vi "configure.vi"(0 "Imaging in":refnum<class "Imaging.lvclass">, 5 "Frame Rate":dbl, 7 "Save Flag Reference":refnum<vi>, 9 "Exposure":dbl, 11 "error in (no error)":errorcluster, 12 "Gain":dbl, 14 "Codec":string) -> (4 "Imaging out":refnum<class "Imaging.lvclass">, 15 "error out":errorcluster)   [LabVIEW 2014, in "Imaging.lvclass"]
uses:
  Imaging.lvclass
  <resource>/objmgr/IMAQImage.rc
  <vilib>/vision/driver/NI_Vision_Acquisition_Software.lvlib
  <vilib>/vision/driver/IMAQdx.llb/IMAQdx Acquisition Mode.ctl
  <vilib>/vision/driver/IMAQdx.llb/IMAQdx Buffer Number Mode.ctl
  <vilib>/vision/Image Controls.llb/IMAQ Image.ctl
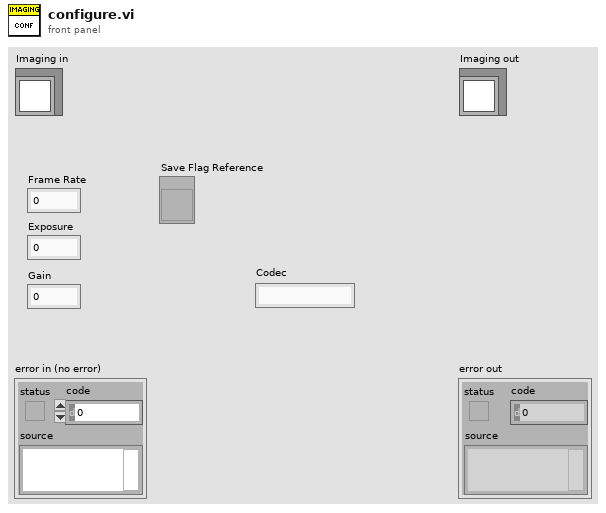
[diagram p1: front panel]
types:
  T1 = typedef "IMAQ Image.ctl" = refnum<image>
  T2 = cluster{"Image Out":T1, dbl, "seconds since 1Jan1904":timestamp}
  T3 = typedef "NI_Vision_Acquisition_Software.lvlib/IMAQdx Buffer Number Mode.ctl" = enum32{"Next", "Last", "Buffer Number", "Every", "Last New"}
  T4 = typedef "NI_Vision_Acquisition_Software.lvlib/IMAQdx Acquisition Mode.ctl" = enum32{"One Shot", "Continuous"}
  T5 = typedef "IMAQdx.ctl" = refnum<k21>
  T6 = typedef "NI_Vision_Acquisition_Software.lvlib/IMAQdx Attribute Type.ctl" = enum32{"U32", "I64", "DBL", "String", "Enum", "Bool", "Command"}
  T7 = cluster{"Attribute Type":T6, "Readable":bool, "Writable":bool, "Attribute Name":string}[]
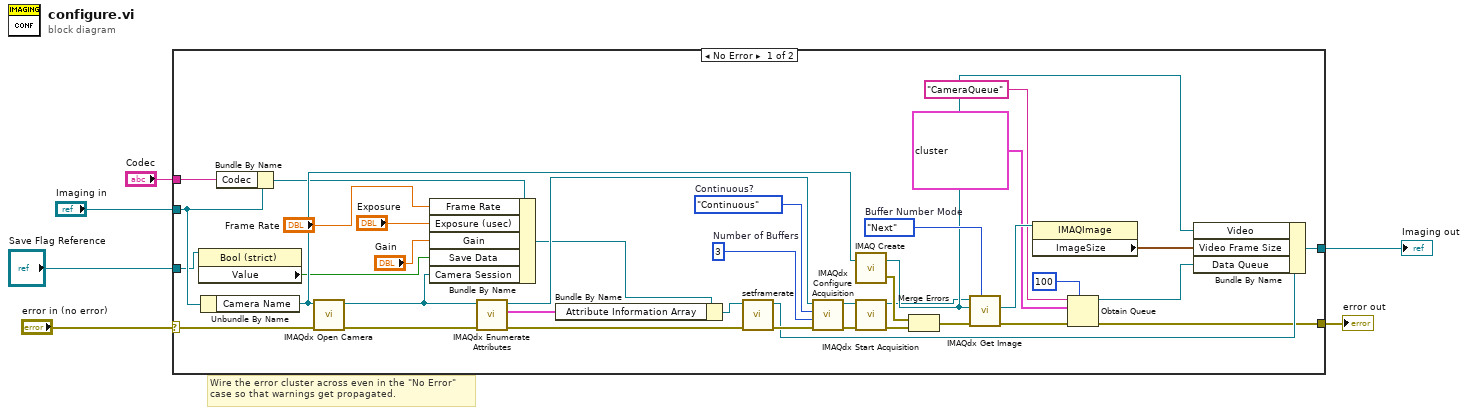
[diagram p0: block diagram]
diagram:
  # "Wire the error cluster across even in the \"No Error\"\ncase so that warnings get propagated."
  n1 = case shown="No Error" "error in (no error)" {
    selector: "error in (no error)" -> [w37 w46]
    tunnel: [w9 w46] -> w5
    tunnel: [w10 w45] -> w3
    tunnel: "Imaging in" -> [w26 w45]
    tunnel: "Codec" -> [w11 _]
    tunnel: "Save Flag Reference" -> [w7 _]
    frame No Error {
      w39 = IMAQdx_Buffer_Number_Mode."Next"  # Buffer Number Mode
      w43 = u32 3  # Number of Buffers
      w44 = IMAQdx_Acquisition_Mode."Continuous"  # Continuous?
      n2 = property class="Bool (strict)"(reference=w7) -> ("Value"=w8:bool)  [unwired: 1 in, 2 out]
      n3 = Unbundle By Name(w26) -> ("Camera Name"=w38:T5)
      n4 = Bundle By Name(cluster=w26, "Codec"=w11) -> (w25:refnum<class "Imaging.lvclass">)
      n5 = call <vilib>:"IMAQdx Open Camera.vi"("error in"=w37, "Session In"=w38) -> ("error out"=w29:errorcluster, "Session Out"=w23:T5)  [unwired: 1 in, 7 out]
      n6 = Bundle By Name(cluster=w25, "Frame Rate"="Frame Rate", "Exposure (usec)"="Exposure", "Gain"="Gain", "Save Data"=w8, "Camera Session"=w23) -> (w20:refnum<class "Imaging.lvclass">)
      n7 = call <vilib>:"IMAQdx Enumerate Attributes.vi"("error in"=w29, "Session In"=w23) -> ("error out"=w18:errorcluster, "Attribute Information Array"=w28:T7, "Session Out"=w21:T5)  [unwired: 7 in]
      n8 = Bundle By Name(cluster=w20, "Attribute Information Array"=w28) -> (w17:refnum<class "Imaging.lvclass">)
      n9 = call-dynamic "setframerate.vi"("error in (no error)"=w18, "Imaging in"=w17) -> ("error out"=w16:errorcluster, "Imaging out"=w15:refnum<class "Imaging.lvclass">)  [unwired: 8 in]
      n10 = call <vilib>:"IMAQdx Configure Acquisition.vi"("error in"=w16, "Number of Buffers"=w43, "Continuous?"=w44, "Session In"=w21) -> ("error out"=w22:errorcluster, "Session Out"=w24:T5)  [unwired: 6 out]
      n11 = call "IMAQ Create"("Image Name"=w38) -> ("New Image"=w36:T1, "error out"=w42:errorcluster)  [unwired: 3 in, 1 out]
      n12 = call <vilib>:"IMAQdx Start Acquisition.vi"("error in"=w22, "Session In"=w24) -> ("error out"=w41:errorcluster, "Session Out"=w19:T5)  [unwired: 8 out]
      n13 = Merge Errors(w42, w41) -> (w14:errorcluster)
      n14 = call <vilib>:"IMAQdx Get Image.vi"("Buffer Number Mode (Next)"=w39, "error in"=w14, "Image In"=w36, "Session In"=w19) -> ("error out"=w27:errorcluster, "Image Out"=w40:T1)  [unwired: 1 in, 5 out]
      n15 = property class="IMAQImage"(reference=w40) -> ("ImageSize"=w35:cluster{"x":i32, "y":i32})  [unwired: 1 in, 2 out]
      n16 = Obtain Queue(max queue size (-1, unlimited)=100, name (unnamed)="CameraQueue", element data type=T2 {"Image Out"=refnum, 0.0, "seconds since 1Jan1904"=timestamp(0 s since 1904-01-01)} ("output cluster"), error in (no error)=w27) -> (queue out=w12:refnum<queue>, error out=w9:errorcluster)  [unwired: 1 in, 1 out]
      n17 = Bundle By Name(cluster=w15, "Video"=w36, "Video Frame Size"=w35, "Data Queue"=w12) -> (w10:refnum<class "Imaging.lvclass">)
    }
    frame Error {
    }
  }
  "error out" <- w5
  "Imaging out" <- w3
